vi "GeneratePieceOfSignal.vi"(6 "#s":dbl=1.0 min=1.0, 8 "noise RMS":dbl=1.0 format="%.2p", 9 "amplitude":dbl, 10 "frequency":dbl=1e-06 min=1e-06, 11 "wfm type":T1) -> (0 "error out":errorcluster, 3 "wfm out":waveform(dbl)(graph))   [LabVIEW 2025]
uses:
  wfm-type.ctl
  <vilib>/express/express analysis/Spectral/Block/exnSpectralBlock spectral measurements PSD poly.vi
  <vilib>/express/express analysis/Spectral/Block/exnSpectralBlock spectral measurements PSD WFM.vi
  <vilib>/express/express analysis/Spectral/XNode/ExpressSpectralMeasurementsBlockNode.xnode
  <vilib>/measure/NI_MABase.lvlib
panel:
  out "x/y":dbl
  out "wfm out 4":waveform(dbl)(graph)
  out "error out 3":errorcluster
  out "wfm out 3":waveform(dbl)(graph)
  out "error out 2":errorcluster
  out "wfm out 2":waveform(dbl)(graph)
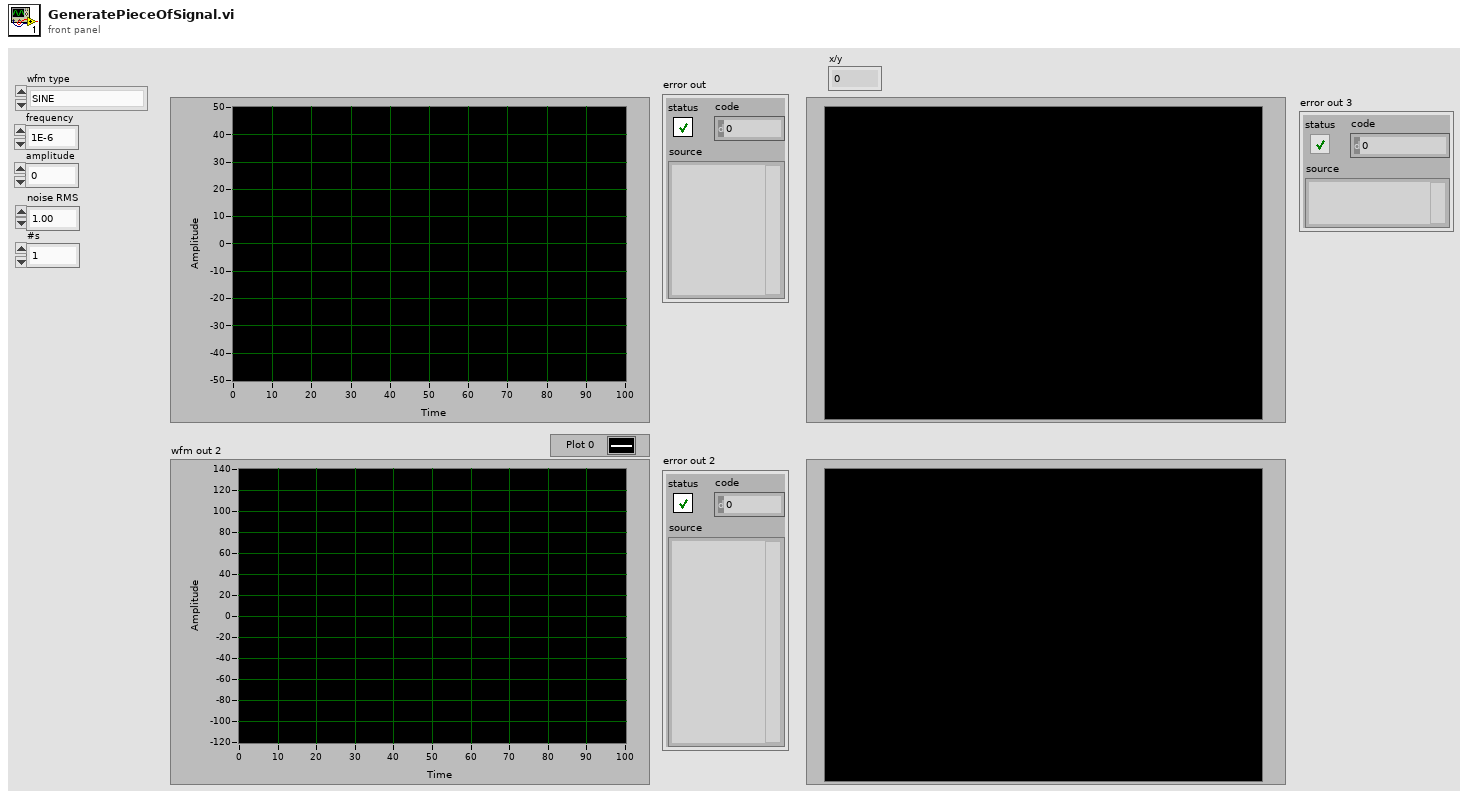
[diagram p1: front panel]
types:
  T1 = typedef "wfm-type.ctl" = enum16{"SINE", "SQUARE", "TRIANGLE", "SAWTOOTH"}
  T2 = cluster{"lower cutoff freq":dbl, "higher cutoff freq":dbl, "order":i32}
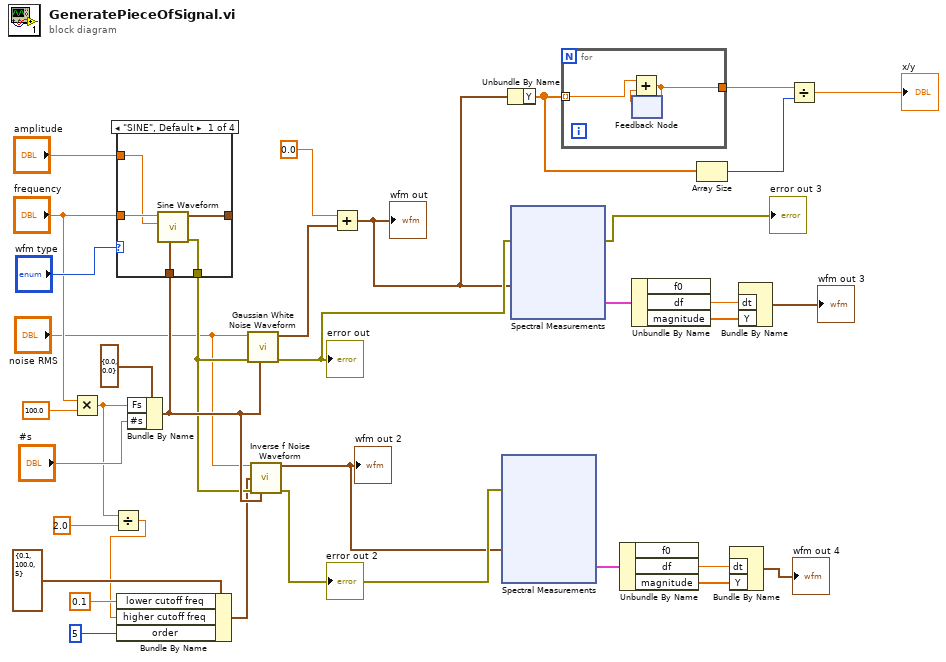
[diagram p0: block diagram]
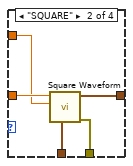
[diagram p2: hidden frame]
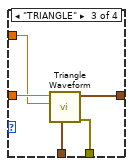
[diagram p3: hidden frame]
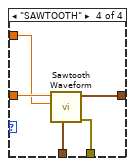
[diagram p4: hidden frame]
diagram:
  n1 = Multiply(x="frequency", y=100.0) -> (x*y=w20:dbl)
  n2 = Divide(x=w20, y=2.0) -> (x/y=w19:dbl)
  n3 = Bundle By Name(cluster=T2 {"lower cutoff freq"=0.1, "higher cutoff freq"=100.0, "order"=5} ("filter specifications"), "lower cutoff freq"=0.1, "higher cutoff freq"=w19, "order"=5) -> (w23:T2)
  n4 = Bundle By Name(cluster=cluster{"Fs":dbl, "#s":dbl} {"Fs"=0.0, "#s"=0.0} ("sampling info"), "Fs"=w20, "#s"="#s") -> (w28:cluster{"Fs":dbl, "#s":dbl})
  n5 = case shown="\"SINE\", Default" "wfm type" {
    tunnel: "frequency" -> [w40 w45 w50 w55]
    tunnel: "amplitude" -> [w39 w44 w49 w54]
    tunnel: [w38 w43 w48 w53] -> w27
    tunnel: w28 -> [w37 w42 w47 w52]
    tunnel: [w36 w41 w46 w51] -> _
    frame "SINE", Default {
      n6 = call <vilib>:"Sine Waveform.vi"("sampling info"=w37, "amplitude"=w39, "frequency"=w40) -> ("error out"=w38:errorcluster, "signal out"=w36:waveform(dbl))  [unwired: 7 in]
    }
    frame "SQUARE" {
      n7 = call <vilib>:"Square Waveform.vi"("sampling info"=w42, "amplitude"=w44, "frequency"=w45) -> ("error out"=w43:errorcluster, "signal out"=w41:waveform(dbl))  [unwired: 7 in]
    }
    frame "TRIANGLE" {
      n8 = call <vilib>:"Triangle Waveform.vi"("sampling info"=w47, "amplitude"=w49, "frequency"=w50) -> ("error out"=w48:errorcluster, "signal out"=w46:waveform(dbl))  [unwired: 7 in]
    }
    frame "SAWTOOTH" {
      n9 = call <vilib>:"Sawtooth Waveform.vi"("sampling info"=w52, "amplitude"=w54, "frequency"=w55) -> ("error out"=w53:errorcluster, "signal out"=w51:waveform(dbl))  [unwired: 7 in]
    }
  }
  n10 = call <vilib>:"Gaussian White Noise Waveform.vi"("sampling info"=w28, "error in (no error)"=w27, "standard deviation"="noise RMS") -> ("error out"=w18:errorcluster, "signal out"=w29:waveform(dbl))  [unwired: 7 in]
  "error out" <- w18
  n11 = call <vilib>:"Inverse f Noise Waveform.vi"("noise density"="noise RMS", "filter specifications"=w23, "error in (no error)"=w27, "sampling info"=w28) -> ("signal out"=w12:waveform(dbl), "error out"=w13:errorcluster)  [unwired: 7 in, 3 out]
  "wfm out 2" <- w12
  "error out 2" <- w13
  n12 = Add(x=0.0, y=w29) -> (x+y=w5:waveform(dbl))
  "wfm out" <- w5
  n13 = xnode "Spectral Measurements"("Signals"=w12, "error in (no error)"=w13) -> ("PSD"=w11:cluster{"f0":dbl, "df":dbl, "magnitude":dbl[]})  [unwired: 1 out]
  n14 = Unbundle By Name(w5) -> ("Y"=w2:dbl[])
  n15 = xnode "Spectral Measurements"("Signals"=w5, "error in (no error)"=w18) -> ("PSD"=w17:cluster{"f0":dbl, "df":dbl, "magnitude":dbl[]}, "error out"=→"error out 3":errorcluster)
  n16 = for {
    tunnel: w2 -> [w58] mode=indexing
    tunnel: [w56] -> w4
    n17 = feedback #1() -> (w57:dbl)  [unwired: 1 in]
    n18 = Add(x=w58, y=w57) -> (x+y=w56:dbl)
    n19 = feedback-in #1(w56) -> ()
  }
  n20 = Unbundle By Name(w11) -> ("df"=w10:dbl, "magnitude"=w9:dbl[])  [unwired: 1 out]
  n21 = Unbundle By Name(w17) -> ("df"=w14:dbl, "magnitude"=w6:dbl[])  [unwired: 1 out]
  n22 = Array Size(array=w2) -> (size(s)=w3:i32)
  n23 = Bundle By Name("dt"=w10, "Y"=w9) -> (→"wfm out 4":waveform(dbl))  [unwired: 1 in]
  n24 = Bundle By Name("dt"=w14, "Y"=w6) -> (→"wfm out 3":waveform(dbl))  [unwired: 1 in]
  n25 = Divide(x=w4, y=w3) -> (x/y=→"x/y":dbl)
